vi "Calculate Cross Spectrum (SubVI).vi"(9 "Center Frequency (Hz)":dbl, 10 "signal in 2":waveform(dbl), 11 "signal in 1":waveform(dbl)) -> (2 "Skew [s]":dbl format="%#_6p", 3 "Frequency (Hz)":dbl format="%#_6p")   [LabVIEW 2021]
uses:
  <vilib>/measure/NI_MAPro.lvlib
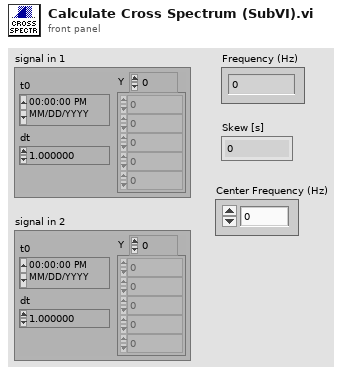
[diagram p1: front panel]
types:
  T1 = cluster{"dB On (F)":bool, "unwrap phase (F)":bool, "convert to degree (F)":bool}
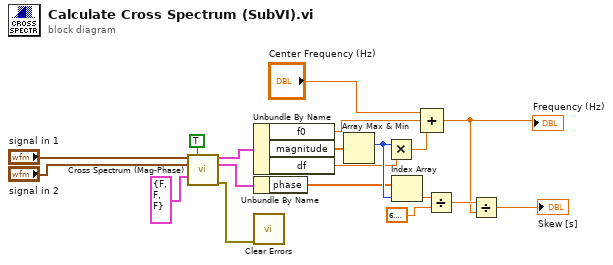
[diagram p0: block diagram]
diagram:
  n1 = call <vilib>:"Cross Spectrum (Mag-Phase).vi"("time signal X"="signal in 1", "restart averaging (F)"=TRUE, "time signal Y"="signal in 2", "view"=T1 {"dB On (F)"=FALSE, "unwrap phase (F)"=FALSE, "convert to degree (F)"=FALSE}) -> ("magnitude"=w7:cluster{"f0":dbl, "df":dbl, "magnitude":dbl[]}, "phase"=w8:cluster{"f0":dbl, "df":dbl, "phase":dbl[]}, "error out"=w6:errorcluster)  [unwired: 7 in, 2 out]
  n2 = Unbundle By Name(w7) -> ("f0"=w4:dbl, "magnitude"=w9:dbl[], "df"=w11:dbl)
  n3 = Unbundle By Name(w8) -> ("phase"=w12:dbl[])
  n4 = call <vilib>:"Clear Errors.vi"("error in (no error)"=w6) -> ()  [unwired: 5 in, 2 out]
  n5 = Array Max & Min(array=w9) -> (max index (indices)=w13:i32)  [unwired: 3 out]
  n6 = Multiply(x=w13, y=w11) -> (x*y=w3:dbl)
  n7 = Index Array(array=w12, index=w13) -> (element=w14:dbl)
  n8 = Compound Arithmetic op=ADD("Center Frequency (Hz)", w4, w3) -> (w2:dbl)
  "Frequency (Hz)" <- w2
  n9 = Divide(x=w14, y=6.283185307179586) -> (x/y=w16:dbl)
  n10 = Divide(x=w16, y=w2) -> (x/y=→"Skew [s]":dbl)
